vi "m10.wf.ramp.vi"(0 "Waveform In":waveform(dbl)={"t0"=timestamp(0 s since 1904-01-01), "dt"=0.0, "Y"=[]}, 5 "Ramp Length (s)":dbl=0.01, 11 "error in (no error)":errorcluster) -> (4 "Waveform Out":waveform(dbl), 15 "error out":errorcluster)   [LabVIEW 2013]
uses:
  <vilib>/Waveform/WDTOps.llb/WDT Waveform Duration DBL.vi
  <vilib>/Waveform/WDTOps.llb/WDT Append Waveforms DBL.vi
  <vilib>/measure/NI_MABase.lvlib
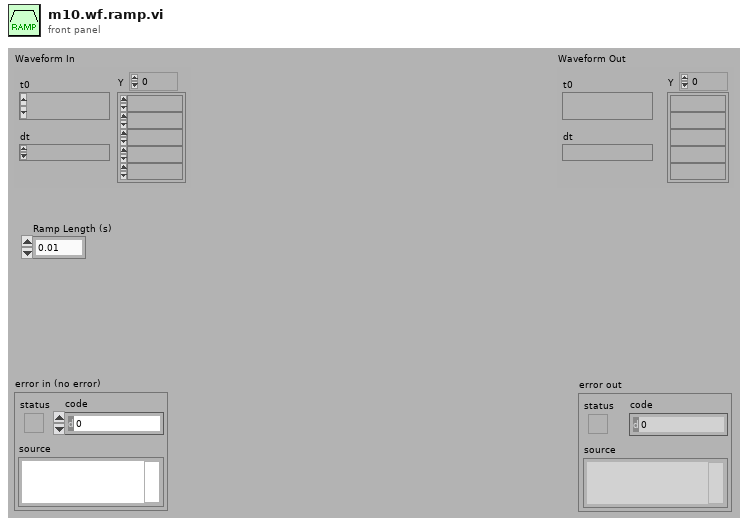
[diagram p1: front panel]
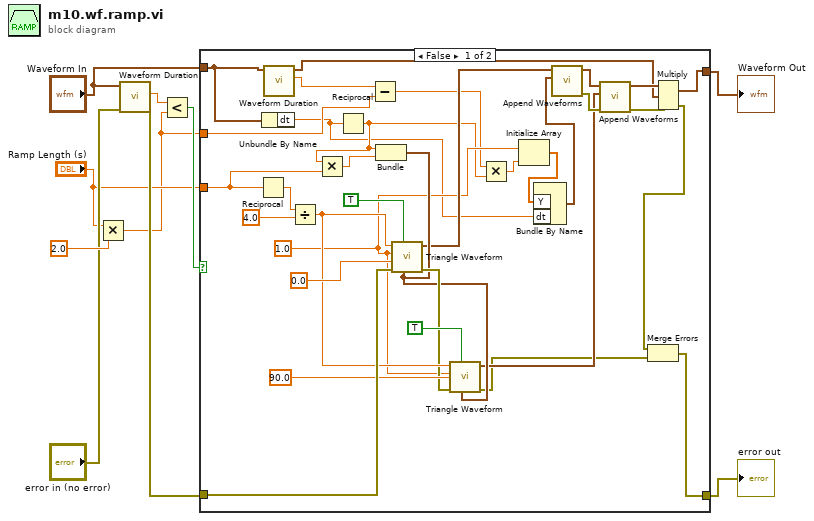
[diagram p0: block diagram]
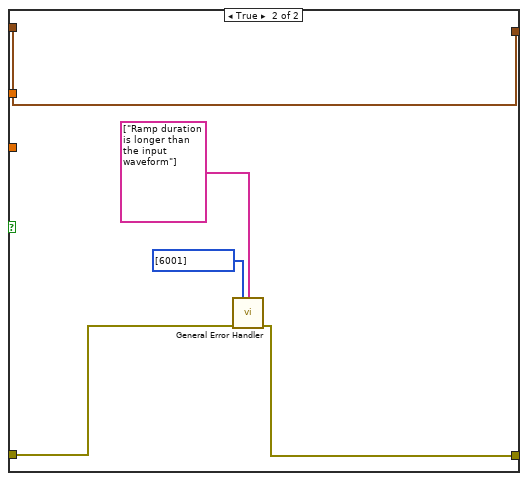
[diagram p2: hidden frame]
diagram:
  n1 = Multiply(x="Ramp Length (s)", y=2.0) -> (x*y=w1:dbl)
  n2 = call-poly <vilib>:"Waveform Duration.vi"("error in (no error)"="error in (no error)", "waveform in"="Waveform In") -> ("error out"=w6:errorcluster, "duration"=w10:dbl)  [unwired: 7 in, 1 out]
  n3 = Less?(x=w10, y=w1) -> (x < y?=w8:bool)
  n4 = case shown="False" w8 {
    tunnel: w6 -> [w40 w48]
    tunnel: [w18 w47] -> w3
    tunnel: "Waveform In" -> [w25 w44]
    tunnel: [w22 w44] -> w4
    tunnel: "Ramp Length (s)" -> [w28 _]
    tunnel: w1 -> [w26 _]
    frame False {
      w15 = 1.0 ("amplitude")
      n5 = Reciprocal(x=w28) -> (1/x=w43:dbl)
      n6 = Unbundle By Name(w25) -> ("dt"=w12:dbl)
      n7 = call-poly <vilib>:"Waveform Duration.vi"("waveform in"=w25) -> ("duration"=w23:dbl, "waveform out"=w24:waveform(dbl))  [unwired: 8 in, 1 out]
      n8 = Divide(x=w43, y=4.0) -> (x/y=w36:dbl)
      n9 = Reciprocal(x=w12) -> (1/x=w13:dbl)
      n10 = Multiply(x=w13, y=w28) -> (x*y=w39:dbl)
      n11 = Subtract(x=w23, y=w26) -> (x-y=w14:dbl)
      n12 = Bundle(w13, w39) -> (w33:cluster{dbl, dbl})  [unwired: 1 in]
      n13 = call <vilib>:"Triangle Waveform.vi"("sampling info"=w33, "reset signal"=TRUE, "error in (no error)"=w40, "phase"=0.0, "amplitude"=w15, "frequency"=w36) -> ("error out"=w34:errorcluster, "signal out"=w31:waveform(dbl))  [unwired: 4 in]
      n14 = call <vilib>:"Triangle Waveform.vi"("sampling info"=w33, "reset signal"=TRUE, "error in (no error)"=w34, "phase"=90.0, "amplitude"=w15, "frequency"=w36) -> ("error out"=w19:errorcluster, "signal out"=w29:waveform(dbl))  [unwired: 4 in]
      n15 = Multiply(x=w14, y=w13) -> (x*y=w16:dbl)
      n16 = Initialize Array(w15, w16) -> (w17:dbl[])
      n17 = Bundle By Name("Y"=w17, "dt"=w12) -> (w11:waveform(dbl))  [unwired: 1 in]
      n18 = call-poly <vilib>:"Append Waveforms.vi"("waveform B"=w11, "waveform A"=w31) -> ("error out"=w30:errorcluster, "waveform out"=w32:waveform(dbl))  [unwired: 8 in]
      n19 = call-poly <vilib>:"Append Waveforms.vi"("error in (no error)"=w30, "waveform B"=w29, "waveform A"=w32) -> ("error out"=w21:errorcluster, "waveform out"=w27:waveform(dbl))  [unwired: 7 in]
      n20 = Multiply(1:w24, 2:w27, 4:w21) -> (0:w22:waveform(dbl), 3:w20:errorcluster)
      n21 = Merge Errors(w20, w19) -> (w18:errorcluster)
    }
    frame True {
      n22 = call <vilib>:"General Error Handler.vi"("[user-defined codes]"=i32[] [6001], "[user-defined descriptions]"=string[] ["Ramp duration is longer than the input waveform"], "error in (no error)"=w48) -> ("error out"=w47:errorcluster)  [unwired: 8 in, 4 out]
    }
  }
  "Waveform Out" <- w4
  "error out" <- w3
